vi "Zadniae_tablice_gotowe.vi"() -> ()   [LabVIEW 2012]
panel:
  out "Wartoœci napiêcia [V] i natê¿enia [A]":dbl[][](array[numeric])
  in  "Losowa wartoœæ napiêcia || Losowa wartoœæ natê¿enia":bool
  in  "Podaj wartoœæ rezystancji [Om]":dbl
  # "Program wyznacza wartoœæ napiêcia i natê¿enia dla zadanej rezystancji na podstawie prawa Ohma i losowych wartoœci napiêcia/natê¿enia"
  # "Wybierz która wartoœæ bêdzie losowana"
  # "Napiêcie"
  # "Natê¿enie"
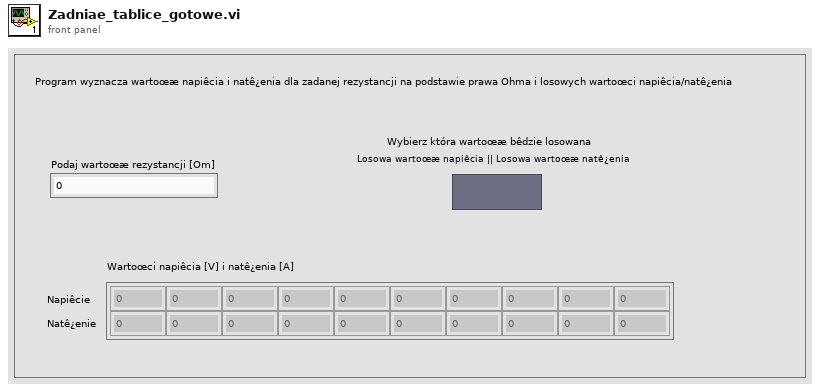
[diagram p1: front panel]
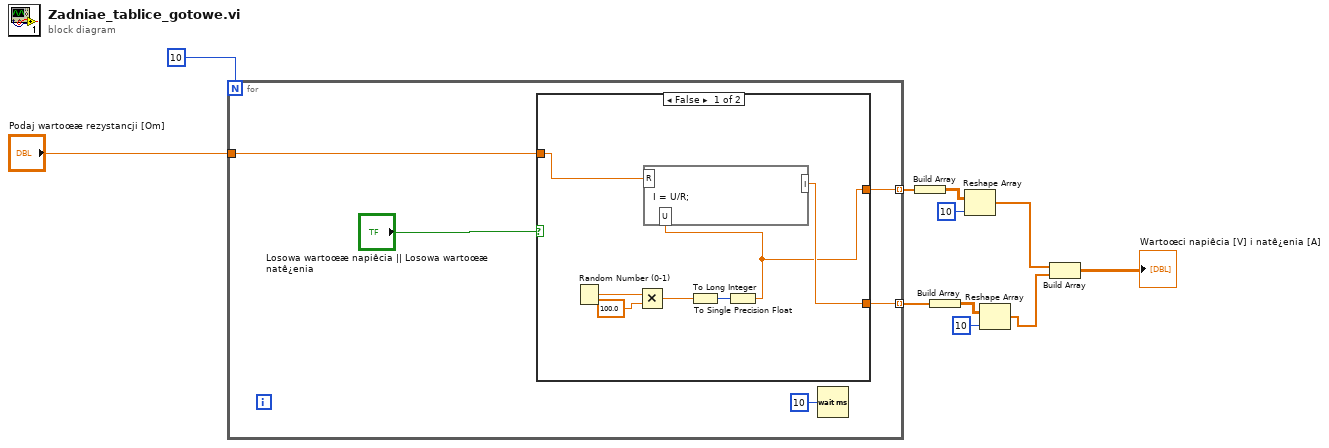
[diagram p0: block diagram]
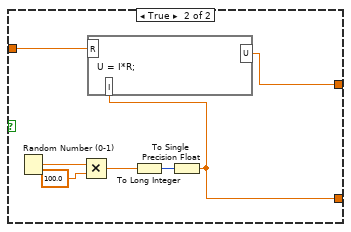
[diagram p2: hidden frame]
diagram:
  n1 = for {
    N: 10 -> [_]
    tunnel: "Podaj wartoœæ rezystancji [Om]" -> [w15]
    tunnel: [w14] -> w5 mode=indexing
    tunnel: [w13] -> w4 mode=indexing
    n2 = case shown="False" "Losowa wartoœæ napiêcia || Losowa wartoœæ natê¿enia" {
      tunnel: w15 -> [w19 w27]
      tunnel: [w17 w26] -> w14
      tunnel: [w18 w24] -> w13
      frame False {
        n3 = Random Number (0-1)() -> (number: 0 to 1=w22:dbl)
        n4 = Multiply(x=w22, y=100.0) -> (x*y=w21:dbl)
        n5 = To Long Integer(number=w21) -> (32bit integer=w20:i32)
        n6 = To Single Precision Float(number=w20) -> (single precision float=w17:sgl)
        n7 = formula code="I = U/R;"("U"=w17, "R"=w19) -> ("I"=w18:dbl)
      }
      frame True {
        n8 = Random Number (0-1)() -> (number: 0 to 1=w29:dbl)
        n9 = Multiply(x=w29, y=100.0) -> (x*y=w28:dbl)
        n10 = To Long Integer(number=w28) -> (32bit integer=w25:i32)
        n11 = To Single Precision Float(number=w25) -> (single precision float=w24:sgl)
        n12 = formula code="U = I*R;"("I"=w24, "R"=w27) -> ("U"=w26:dbl)
      }
    }
    n13 = Wait (ms)(milliseconds to wait=u32 10) -> ()  [unwired: 1 out]
  }
  n14 = Build Array(w5) -> (w11:dbl[][])
  n15 = Build Array(w4) -> (w9:dbl[][])
  n16 = Reshape Array(w11, 10 ("dimension size")) -> (w3:dbl[])
  n17 = Reshape Array(w9, 10 ("dimension size")) -> (w1:dbl[])
  n18 = Build Array(w3, w1) -> (→"Wartoœci napiêcia [V] i natê¿enia [A]":dbl[][])
